vi "Quick Start - Complete Streaming.vi"() -> ()   [LabVIEW 2020]
uses:
  Nominal Client/Nominal Client.lvclass/Nominal Client.ctl
  8bc873d6-11f2-47b8-afa9-2ee06eb45ce7.vi
  68912467-c1c9-4a94-a3ad-dccbebf4617c.vi
  6412a388-4fe4-4984-8121-4c3d8e6ce4ff.vi
  Nominal Client/private_data.set.vi
  6412a388-4fe4-4984-8121-4c3d8e6ce4ff.vi/cdde0a50-1f2d-45b6-8c5c-67b334d1f5bb.vi
  6412a388-4fe4-4984-8121-4c3d8e6ce4ff.vi/2aaf4cd1-b7d0-4e89-be55-e948b2020e34.vi
  <vilib>/LabVIEW Open Source Project/Epoch Date & Time/epoch.UNIX/Epoch.UNIX.lvclass
  C:/Program Files/National Instruments/LabVIEW 2020/vi.lib/LabVIEW Open Source Project/Epoch Date & Time/epoch/Epoch.lvclass
  <vilib>/Utility/file.llb/Application Directory.vi
  <vilib>/Utility/error.llb/Error Cluster From Error Code.vi
  <vilib>/addons/_JKI.lib/REST Client/classes/REST Client/Create REST Client.vi
  <vilib>/LabVIEW Open Source Project/Epoch Date & Time/Get Epoch Time.vi
  <vilib>/JDP Science/JSONtext/Variant to JSON Text.vi
  <vilib>/JDP Science/JSONtext/Array of Variants to JSON Object.vi
  <vilib>/JDP Science/JSONtext/Set Item.vi
  Nominal Client/http.post.vi
  Nominal Client/Nominal Client.lvclass
  <vilib>/addons/_JKI.lib/REST Client/classes/REST Client/REST Client.lvclass
  <vilib>/JDP Science/JSONtext/LVClass Serializer/JSONtext LVClass Serializer.lvclass
panel:
  out "response":T1
  out "Created Data Source":T2
  in  "API Token":string
  in  "Stop":bool
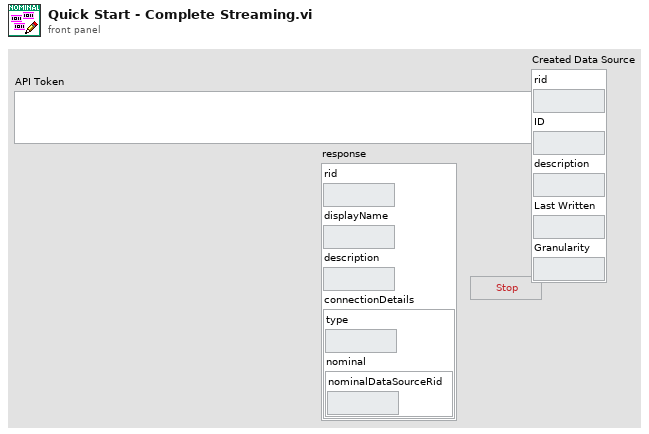
[diagram p1: front panel]
types:
  T1 = cluster{"rid":string, "displayName":string, "description":string, "connectionDetails":cluster{"type":string, "nominal":cluster{"nominalDataSourceRid":string}}}
  T2 = cluster{"rid":string, "ID":string, "description":string, "Last Written":string, "Granularity":string}
  T3 = cluster{"channel":string, "current time":timestamp, "data":dbl}
  T4 = cluster{"[0]":refnum<queue>, "[1]":refnum<queue>, "[2]":refnum<queue>}
  T5 = cluster{"channel":string, "current time":timestamp, "data":dbl}[]
  T6 = cluster{"UNIX Timestamp":cluster{"Seconds":i64, "Nanoseconds":i64}, "data":dbl}
  T7 = cluster{"channel":string, cluster{"UNIX Timestamp":cluster{"Seconds":i64, "Nanoseconds":i64}, "data":dbl}[]}
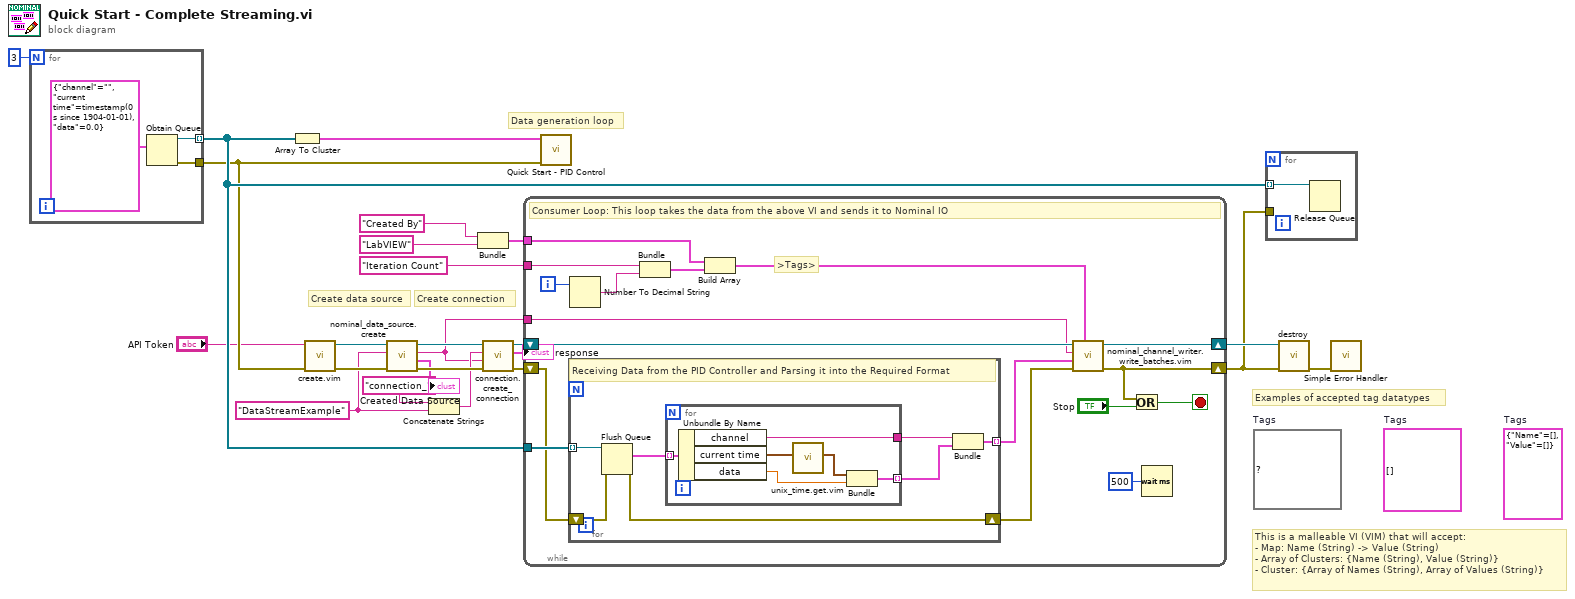
[diagram p0: block diagram]
diagram:
  w4 = "DataStreamExample" ("Name")
  (unwired) cluster{"Name":string, "Value":string}[] []  # Tags
  (unwired) cluster{"Name":string[], "Value":string[]} {"Name"=[], "Value"=[]}  # Tags
  (unwired) map{string, string} {}  # Tags
  # "Create connection"
  # "Create data source"
  # "Examples of accepted tag datatypes"
  # "This is a malleable VI (VIM) that will accept:\n- Map: Name (String) -> Value (String)\n- Array of Clusters: {Name (String), Value (String)}\n- Cluster: {Array of Names (String), Array of Values (String)}"
  # "Data generation loop"
  n1 = for {
    N: 3 -> [_]
    tunnel: [w26] -> w21 mode=indexing
    tunnel: [w25] -> w18
    n2 = Obtain Queue(element data type=T3 {"channel"="", "current time"=timestamp(0 s since 1904-01-01), "data"=0.0}) -> (queue out=w26:refnum<queue>, error out=w25:errorcluster)  [unwired: 4 in, 1 out]
  }
  n3 = Array To Cluster(array=w21) -> (cluster=w19:T4)
  n4 = call "create.vim"("error in"=w18, "API Token (string or path)"="API Token") -> ("error out"=w12:errorcluster, "Nominal Client"=w13:refnum<class "Nominal Client.lvclass">)  [unwired: 8 in]
  n5 = call "nominal_data_source.create.vi"("error in"=w12, "Name"=w4, "Nominal Client in"=w13) -> ("error out"=w11:errorcluster, "Created Data Source"=→"Created Data Source":T2, "rid"=w5:string, "Nominal Client out"=w10:refnum<class "Nominal Client.lvclass">)  [unwired: 5 in]
  n6 = Concatenate Strings("connection_" ("string"), w4) -> (w8:string)
  n7 = Bundle("Created By", "LabVIEW") -> (w14:cluster{string, string})  [unwired: 1 in]
  n8 = call "connection.create_connection.vi"("error in"=w11, "nominalDataSourceRid"=w5, "name"=w8, "Nominal Client in"=w10) -> ("error out"=w7:errorcluster, "response"=→"response":T1, "Nominal Client out"=w6:refnum<class "Nominal Client.lvclass">)  [unwired: 4 in, 1 out]
  n9 = while {
    tunnel: w21 -> [w41]
    shift-right: [w37] -> w20
    shift-left: w7 -> [w40]
    shift-right: [w38] -> w24
    shift-left: w6 -> [w39]
    tunnel: "Iteration Count" -> [w32]
    tunnel: w14 -> [w31]
    tunnel: w5 -> [w28]
    i -> [w34]
    stop <- w43 stop-if-true
    # ">Tags>"
    # "Consumer Loop: This loop takes the data from the above VI and sends it to Nominal IO"
    n10 = for {
      tunnel: w41 -> [w51] mode=indexing
      tunnel: [w47] -> w35 mode=indexing
      shift-right: [w45] -> w36
      shift-left: w40 -> [w46]
      # "Receiving Data from the PID Controller and Parsing it into the Required Format"
      n11 = Flush Queue(queue=w51, error in (no error)=w46) -> (remaining elements=w50:T5, error out=w45:errorcluster)  [unwired: 1 out]
      n12 = for {
        tunnel: w50 -> [w57] mode=indexing
        tunnel: [w53] -> w48 mode=indexing
        tunnel: [w52] -> w49
        n13 = Unbundle By Name(w57) -> ("channel"=w52:string, "current time"=w56:timestamp, "data"=w54:dbl)
        n14 = call "unix_time.get.vim"("Time Stamp (empty: now) [single or array]"=w56) -> ("UNIX Timestamp"=w55:cluster{"Seconds":i64, "Nanoseconds":i64})  [unwired: 10 in]
        n15 = Bundle("UNIX Timestamp"=w55, "data"=w54) -> (w53:T6)  [unwired: 1 in]
      }
      n16 = Bundle("channel"=w49, w48) -> (w47:T7)  [unwired: 1 in]
    }
    n17 = Number To Decimal String(number=w34) -> (decimal integer string=w33:string)  [unwired: 1 in]
    n18 = Bundle(w32, w33) -> (w30:cluster{string, string})  [unwired: 1 in]
    n19 = Build Array(w31, w30) -> (w29:cluster{string, string}[])
    n20 = call "nominal_channel_writer.write_batches.vim"("Tags"=w29, "error in"=w36, "batches"=w35, "Data Source RID"=w28, "Nominal Client in"=w39) -> ("error out"=w37:errorcluster, "Nominal Client out"=w38:refnum<class "Nominal Client.lvclass">)  [unwired: 4 in, 1 out]
    n21 = Or(x=w37, y="Stop") -> (x .or. y?=w43:bool)
    n22 = Wait (ms)(milliseconds to wait=u32 500) -> ()  [unwired: 1 out]
  }
  n23 = call "Quick Start - PID Control.vi"("error in (no error)"=w18, "Data"=w19) -> ()  [unwired: 10 in]
  n24 = for {
    tunnel: w21 -> [w58] mode=indexing
    tunnel: w20 -> [_]
    n25 = Release Queue(queue=w58) -> ()  [unwired: 2 in, 3 out]
  }
  n26 = call "destroy.vi"("error in"=w20, "Nominal Client"=w24) -> ("error out"=w23:errorcluster)  [unwired: 9 in]
  n27 = call <vilib>:"Simple Error Handler.vi"("error in (no error)"=w23) -> ()  [unwired: 4 in, 5 out]
